vi "Set Controls.vi"(8 "error in (no error)":errorcluster caption="entrée d'erreur (pas d'erreur)", 11 "UI Cam Basler en entrée":refnum<class "UI Cam Basler.lvclass">) -> (0 "error out":errorcluster caption="sortie d'erreur", 3 "UI Cam Basler en sortie":refnum<class "UI Cam Basler.lvclass">)   [LabVIEW 2023, in "UI Cam Basler.lvclass"]
uses:
  UI Cam Basler.lvclass
  <vilib>/userDefined/High Color/IMAQdx.ctl
  UI Cam Basler.lvclass/UI Cam Basler.ctl
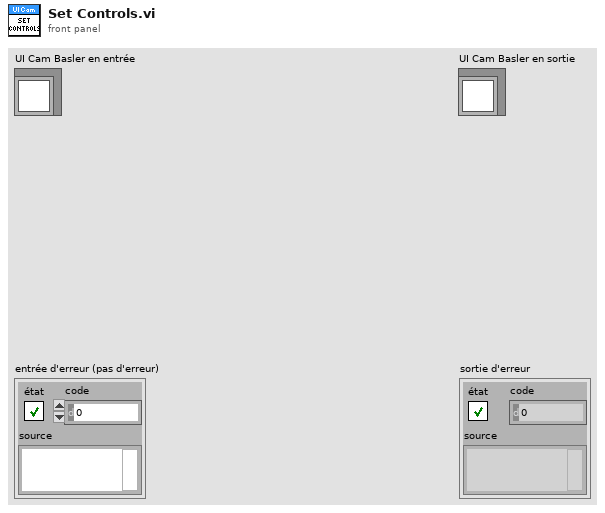
[diagram p1: front panel]
types:
  T1 = typedef "IMAQdx.ctl" = refnum<k21>
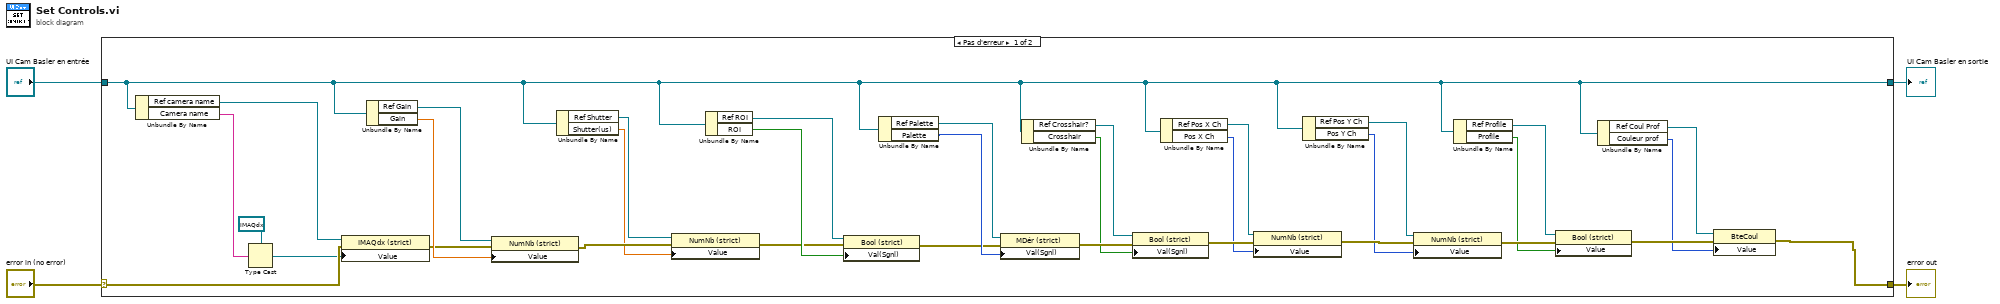
[diagram p0: block diagram]
diagram:
  n1 = case shown="Pas d'erreur" "error in (no error)" {
    selector: "error in (no error)" -> [w38 w40]
    tunnel: [w12 w40] -> w3
    tunnel: [w9 w39] -> w1
    tunnel: "UI Cam Basler en entrée" -> [w9 w39]
    frame No Error {
      n2 = Unbundle By Name(w9) -> ("Ref camera name"=w35:refnum<vi>, "Camera name"=w37:string)
      n3 = Type Cast(type=T1 refnum ("Camera Name"), x=w37) -> (*(type *) &x=w34:T1)
      n4 = property class="IMAQdx (strict)"(reference=w35, error in=w38, "Value"=w34) -> (error out=w31:errorcluster)  [unwired: 1 out]
      n5 = Unbundle By Name(w9) -> ("Ref Gain"=w33:refnum<vi>, "Gain"=w32:dbl)
      n6 = property class="NumNb (strict)"(reference=w33, error in=w31, "Value"=w32) -> (error out=w30:errorcluster)  [unwired: 1 out]
      n7 = Unbundle By Name(w9) -> ("Ref Shutter"=w29:refnum<vi>, "Shutter(us)"=w28:dbl)
      n8 = property class="NumNb (strict)"(reference=w29, error in=w30, "Value"=w28) -> (error out=w25:errorcluster)  [unwired: 1 out]
      n9 = Unbundle By Name(w9) -> ("Ref ROI"=w27:refnum<vi>, "ROI"=w26:bool)
      n10 = property class="Bool (strict)"(reference=w27, error in=w25, "Val(Sgnl)"=w26) -> (error out=w22:errorcluster)  [unwired: 1 out]
      n11 = Unbundle By Name(w9) -> ("Ref Palette"=w24:refnum<vi>, "Palette"=w23:u32)
      n12 = property class="MDér (strict)"(reference=w24, error in=w22, "Val(Sgnl)"=w23) -> (error out=w21:errorcluster)  [unwired: 1 out]
      n13 = Unbundle By Name(w9) -> ("Ref Crosshair?"=w18:refnum<vi>, "Crosshair"=w17:bool)
      n14 = property class="Bool (strict)"(reference=w18, error in=w21, "Val(Sgnl)"=w17) -> (error out=w20:errorcluster)  [unwired: 1 out]
      n15 = Unbundle By Name(w9) -> ("Ref Pos X Ch"=w16:refnum<vi>, "Pos X Ch"=w15:u32)
      n16 = property class="NumNb (strict)"(reference=w16, error in=w20, "Value"=w15) -> (error out=w19:errorcluster)  [unwired: 1 out]
      n17 = Unbundle By Name(w9) -> ("Ref Pos Y Ch"=w14:refnum<vi>, "Pos Y Ch"=w13:u32)
      n18 = property class="NumNb (strict)"(reference=w14, error in=w19, "Value"=w13) -> (error out=w10:errorcluster)  [unwired: 1 out]
      n19 = Unbundle By Name(w9) -> ("Ref Profile"=w8:refnum<vi>, "Profile"=w7:bool)
      n20 = property class="Bool (strict)"(reference=w8, error in=w10, "Value"=w7) -> (error out=w11:errorcluster)  [unwired: 1 out]
      n21 = Unbundle By Name(w9) -> ("Ref Coul Prof"=w5:refnum<vi>, "Couleur prof"=w6:u32)
      n22 = property class="BteCoul"(reference=w5, error in=w11, "Value"=w6) -> (error out=w12:errorcluster)  [unwired: 1 out]
    }
    frame Error {
    }
  }
  "error out" <- w3
  "UI Cam Basler en sortie" <- w1
